vi "01a-add_two_numbers.vi"() -> ()   [LabVIEW 2018, in "LV2Julia_examples.lvlib"]
uses:
  LV2Julia_examples.lvlib
  LV2Julia_core/VIs/Server or client state.ctl
  LV2Julia_core/VIs/detailed error info.ctl
  LV2Julia_core/VIs/StackFrame.ctl
  LV2Julia_core/VIs/Commands.ctl
  a521f879-d34e-4576-958d-ff4dfcea3e86.vi
  be4745b6-8471-45fc-b8a0-8968ce92ea4b.vi
  5a89c37d-8165-4bab-9232-2165bf484997.vi
  <vilib>/Utility/High Resolution Relative Seconds.vi
  be4745b6-8471-45fc-b8a0-8968ce92ea4b.vi/8746a0b0-62a3-40e4-b825-12f6a6230e6b.vi
  be4745b6-8471-45fc-b8a0-8968ce92ea4b.vi/8746a0b0-62a3-40e4-b825-12f6a6230e6b.vi/bc5cf7f8-6c1d-422b-a75d-56be8edab9d2.vi
  be4745b6-8471-45fc-b8a0-8968ce92ea4b.vi/8746a0b0-62a3-40e4-b825-12f6a6230e6b.vi/5a03331b-8486-4786-b5f6-3e60c4d89549.vi
  be4745b6-8471-45fc-b8a0-8968ce92ea4b.vi/8746a0b0-62a3-40e4-b825-12f6a6230e6b.vi/01f183cb-4274-4392-9f55-536a6e5cb750.vi
  LV2Julia_core/VIs/jl-scripts path.vi
  LV2Julia_core/VIs/check ID validity.vi
  LV2Julia_core/VIs/bindata_descr to JSON.vi
  LV2Julia_core/VIs/check cluster field names.vi
  LV2Julia_core/VIs/concat JSON.vi
  LV2Julia_core/VIs/build request.vi
  LV2Julia_core/VIs/Parse server response.vi
  LV2Julia_core/VIs/log jl exceptions.vi
  LV2Julia_core/LV2Julia_core.lvlib
panel:
  out "call duration (ms)":dbl format="%#.2f"
  in  "summands":cluster{"x":dbl, "y":dbl}={"x"=2.0, "y"=2.0}
  in  "next":bool
  out "x+y":dbl=nan
  out "detailed error info":T1
  out "current error":errorcluster
  out "final error":errorcluster
  out "short err code":u8
  in  "stop":bool
  out "ZMQ timeout":bool
  out "Julia script file path":path
  out "temporary script path":path
  out "Jl Server state":T3
  # "After the Julia server started (Jl Server state changed to \"running\", also see the Windows command line window), click onto  Next to get the calculation result. Click onto stop to  stop this VI as well as the Julia server.\n\nNote that the first call of a Julia function may take a fraction of second due to JIT compilation"
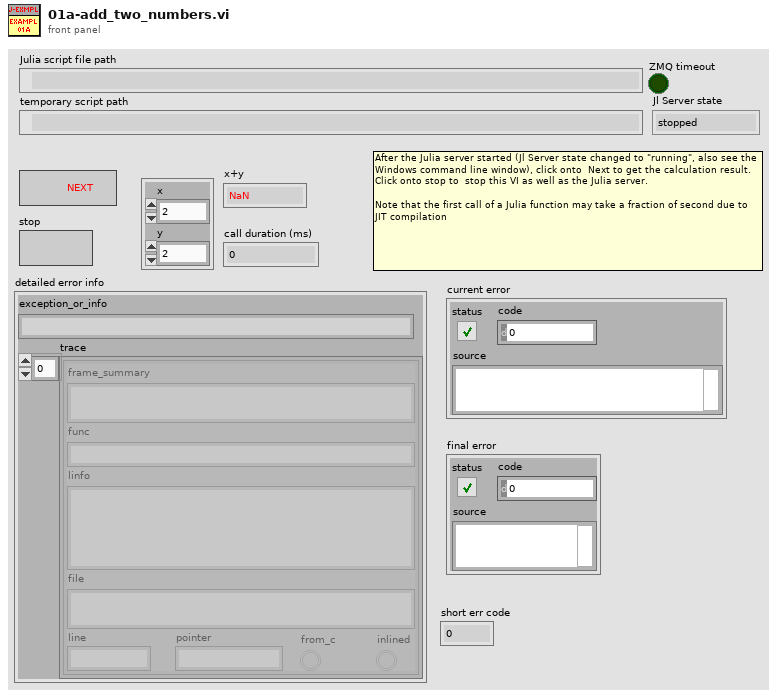
[diagram p1: front panel]
types:
  T1 = typedef "LV2Julia_core.lvlib/detailed error info.ctl" = cluster{"exception_or_info":string, "trace":T2[]}
  T2 = typedef "LV2Julia_core.lvlib/StackFrame.ctl" = cluster{"frame_summary":string, "func":string, "linfo":string, "file":string, "line":i32, "pointer":u64, "from_c":bool, "inlined":bool}
  T3 = typedef "LV2Julia_core.lvlib/Server or client state.ctl" = enum16{"stopped", "running", "unknown"}
  T4 = typedef "LV2Julia_core.lvlib/Commands.ctl" = enum16{"Start Jl-server & Init LV-client", "Send request & Get response ", "Stop Jl-server & Cleanup LV-client", "Cleanup LV-client", "Start Jl-server", "Stop Jl-server", "Init LV-Client", "Cleanup LV-Client", "(not allowed)", "Set LV Client state", "Set Jl Server state", "set ZMQ timeout", "read ZMQ timeout", "read-out state"}
  T5 = typedef "Server state info.ctl" = cluster{"detailed error info":T1, "return code":u8, "Jl Server state":T3}
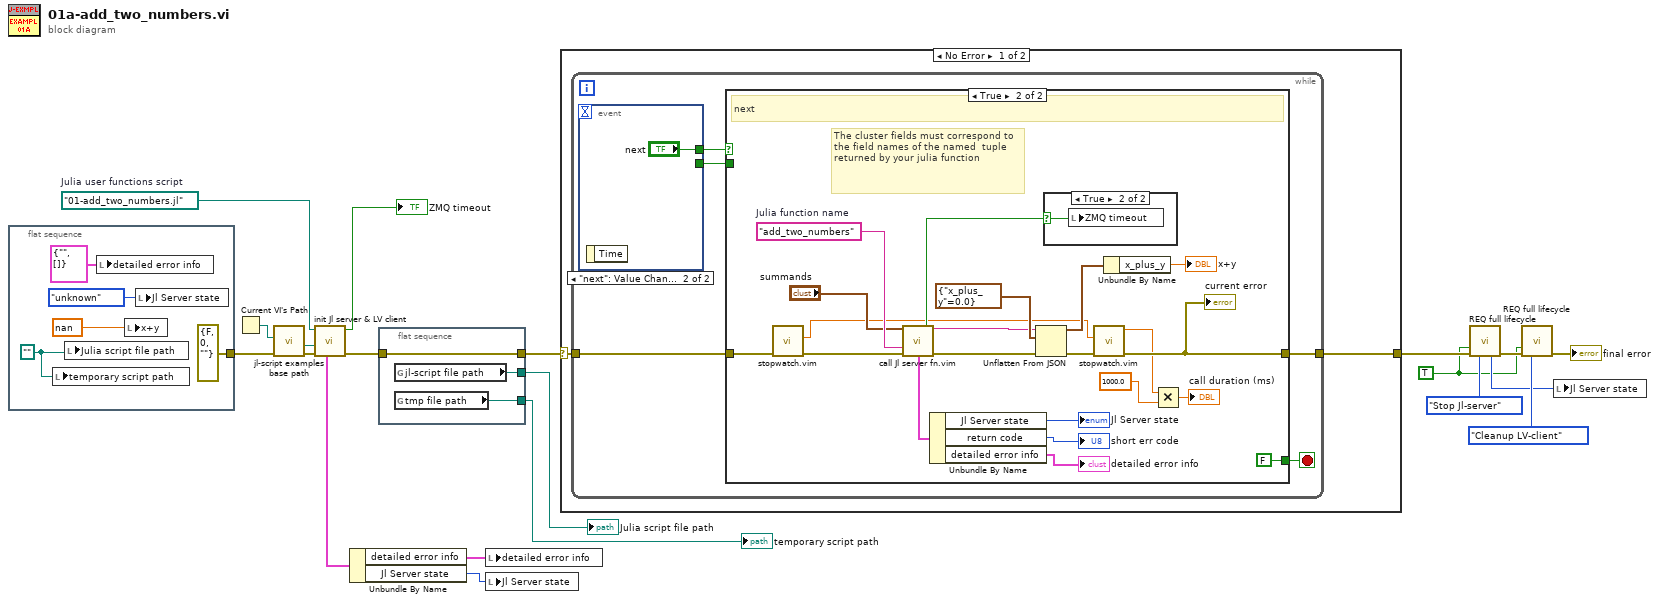
[diagram p0: block diagram]
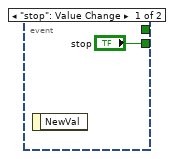
[diagram p2: hidden frame]
diagram:
  w11 = path "01-add_two_numbers.jl"  # Julia user functions script
  w10 = TRUE ("Force command")
  n1 = flat-sequence {
    tunnel: [errorcluster {"status"=FALSE, "code"=0, "source"=""} ("error in (no error)")] -> w7
    frame #0 {
      w21 = path ""
      n2 = local write "temporary script path"(w21) -> ()
      n3 = local write "Julia script file path"(w21) -> ()
      n4 = local write "detailed error info"(T1 {"exception_or_info"="", "trace"=[]} ("detailed error info")) -> ()
      n5 = local write "x+y"(nan ("Server response")) -> ()
      n6 = local write "Jl Server state"(Server_or_client_state."unknown" ("Jl Server state out")) -> ()
    }
  }
  n7 = Current VI's Path() -> (path=w4:path)
  n8 = call "jl-script examples base path.vi"("error in (no error)"=w7, "calling example VI path"=w4) -> ("error out"=w6:errorcluster, "jl-script-examples base path"=w5:path)  [unwired: 8 in]
  n9 = call "init Jl server & LV client.vi"("error in (no error)"=w6, "Base path (not a path)"=w5, "Julia user functions script"=w11) -> ("error out"=w8:errorcluster, "timeout?"=→"ZMQ timeout":bool, "Server state info"=w3:T5)  [unwired: 5 in, 1 out]
  n10 = Unbundle By Name(w3) -> ("detailed error info"=w2:T1, "Jl Server state"=w1:T3)
  n11 = flat-sequence {
    tunnel: [w28] -> w15
    tunnel: w8 -> [w28]
    tunnel: [w27] -> w13
    tunnel: [w26] -> w14
    frame #0 {
      n12 = global read "jl-scripts path.vi" "jl-script file path"() -> (w27:path)
      n13 = global read "jl-scripts path.vi" "tmp file path"() -> (w26:path)
    }
  }
  n14 = local write "detailed error info"(w2) -> ()
  n15 = local write "Jl Server state"(w1) -> ()
  n16 = case shown="No Error" w15 {
    selector: w15 -> [w29 w62]
    tunnel: [w30 w62] -> w20
    frame No Error {
      n17 = while {
        tunnel: w29 -> [w34]
        tunnel: [w35] -> w30
        stop <- w32 stop-if-true
        n18 = event shown="[1] \"next\": Value Change" {
          selector: _ -> [_ _]
          dyn-events: _ -> [_ _]
          timeout: _ -> [_ _]
          tunnel: [_ "next"] -> w33
          tunnel: ["stop" _] -> w31
          event "stop": Value Change {
            n19 = event-data() -> ()  [unwired: 1 in, 1 out]
          }
          event "next": Value Change {
            n20 = event-data() -> ()  [unwired: 1 in, 1 out]
          }
        }
        n21 = case shown="True" w33 {
          tunnel: [w39 w46] -> w35
          tunnel: w34 -> [w39 w50]
          tunnel: [w38 FALSE ("stop this VI only")] -> w32
          tunnel: w31 -> [w38 _]
          frame False {
            # "stop"
          }
          frame True {
            w57 = "add_two_numbers"  # Julia function name
            # "The cluster fields must correspond to the field names of the named  tuple returned by your julia function"
            # "next"
            n22 = call "stopwatch.vim"("anything in"=w50) -> ("copy of anything out"=w49:errorcluster, "current timepoint"=w45:dbl)  [unwired: 8 in, 1 out]
            n23 = call "call Jl server fn.vim"("Arguments 1"="summands", "fun2call"=w57, "error in (no error)"=w49) -> ("timeout?"=w56:bool, "JSON received"=w54:string, "Server state info"=w43:T5, "error out"=w55:errorcluster)  [unwired: 8 in, 1 out]
            n24 = Unbundle By Name(w43) -> ("Jl Server state"=→"Jl Server state":T3, "return code"=→"short err code":u8, "detailed error info"=→"detailed error info":T1)
            n25 = Unflatten From JSON(JSON string=w54, type and defaults=cluster{"x_plus_y":dbl} {"x_plus_y"=0.0} ("parsed response"), error in (no error)=w55) -> (value=w48:cluster{"x_plus_y":dbl}, error out=w47:errorcluster)  [unwired: 4 in]
            n26 = case shown="True" w56 {
              selector: w56 -> [_ w61]
              frame False {
              }
              frame True {
                n27 = local write "ZMQ timeout"(w61) -> ()
              }
            }
            n28 = call "stopwatch.vim"("anything in"=w47, "prev timepoint (0)"=w45) -> ("copy of anything out"=w46:errorcluster, "delta t (s)"=w44:dbl)  [unwired: 7 in, 1 out]
            "current error" <- w46
            n29 = Unbundle By Name(w48) -> ("x_plus_y"=→"x+y":dbl)
            n30 = Multiply(x=w44, y=1000.0) -> (x*y=→"call duration (ms)":dbl)
          }
        }
      }
    }
    frame Error {
    }
  }
  n31 = call "REQ full lifecycle.vi"("Force command"=w10, "error in"=w20, "command"=Commands."Stop Jl-server") -> ("Jl Server state out"=w12:T3, "error out"=w18:errorcluster)  [unwired: 6 in, 5 out]
  n32 = call "REQ full lifecycle.vi"("Force command"=w10, "error in"=w18, "command"=Commands."Cleanup LV-client") -> ("error out"=→"final error":errorcluster)  [unwired: 6 in, 6 out]
  n33 = local write "Jl Server state"(w12) -> ()
  "temporary script path" <- w14
  "Julia script file path" <- w13
